vi "HEWH RLT PRAT.vi"() -> ()   [LabVIEW 2023] (continued)
            n274 = Unbundle By Name(w837) -> ("Core HEWH Data Input A.Module 4 Relay Status.Intellifaucet (% Open)"=w836:dbl, "Core HEWH Data Input A.Module 4 Relay Status.Proportioning Valve (%Open)"=w835:dbl, "Core HEWH Data Input A.Module 4 Relay Status.Intellifaucet Temp Setpoint (F)"=w834:dbl)
            n275 = local write "Valve % Open"(w836) -> ()
            n276 = local write "Proportioning\nValve"(w835) -> ()
            n277 = local write "Temp (°F)"(w834) -> ()
            n278 = call <vilib>:"Add State(s) to Queue__jki_lib_state_machine.vi"("State(s) in (\"\")"=w840) -> ("States Out"=w839:string)  [unwired: 14 in]
          }
          frame "Update File Locations" {
            n279 = flat-sequence {
              tunnel: w845 -> [w856]
              tunnel: w843 -> [w855]
              tunnel: w847 -> [w854]
              tunnel: w842 -> [w853]
              tunnel: w841 -> [w852]
              tunnel: [w851] -> w846
              tunnel: w846 -> [w857]
              tunnel: [w857] -> w844
              frame #0 {
                n280 = Bundle By Name(cluster=w856, "File Locations A"=w855, "File Locations B"=w854, "File Locations C"=w853, "File Locations D"=w852) -> (w851:T88)
              }
              frame #1 {
                n281 = Unbundle By Name(w857) -> ("Core HEWH Data Input A"=w861:T13, "Core HEWH Data Input B"=w860:T13, "Core HEWH Data Input C"=w859:T13, "Core HEWH Data Input D"=w858:T13)
                n282 = local write "Core HEWH Data Input B"(w860) -> ()
                n283 = local write "Core HEWH Data Input A"(w861) -> ()
                n284 = local write "Core HEWH Data Input C"(w859) -> ()
                n285 = local write "Core HEWH Data Input D"(w858) -> ()
              }
              frame #2 {
                "Start Draw Loop" <- TRUE ("Init Complete")
              }
            }
            n286 = call <vilib>:"Add State(s) to Queue__jki_lib_state_machine.vi"("State(s) in (\"\")"=w850) -> ("States Out"=w849:string)  [unwired: 14 in]
          }
          frame "Load Configuration" {
            w866 = u16 502 ("Test Fixture Hardware.ITHX-Temp Humidity.Remote Port")
            w875 = T89 {"Test Fixture Hardware"={"Power "={"Yokogawa"={"WT210"={"Sample Rate (1: 0.25s)"=0, "A Range (12: 20A)"=0, "V Range (6: 600V)"=0, "Power VISA Yokogawa WT210"=""}, "WT500"={"Power VISA Yokogawa WT500"="", "V Range (8: 1000V)"=0, "I Range (7: 40A)"=0, "Update Rate (3: 500ms)"=0}, "WT310_2"={"Sample Rate (1: 0.25s)"=0, "A Range (12: 20A)"=0, "V Range (6: 600V)"=0, "Power VISA Yokogawa WT310_2"=""}, "WT310_3"={"Sample Rate (1: 0.25s)"=0, "A Range (12: 20A)"=0, "V Range (6: 600V)"=0, "Power VISA Yokogawa WT310_3"=""}}, "Aplus"={"Aplus IP Address"="", "Remote Port"=0, "Instrument"="", "Instr Driver Revision"=""}, "Power Limits"={"Crest Factor"={"Upper Limit"=0.0, "Lower Limit"=0.0}, "Harmonic Content"={"Uthd"=0.0}, "Voltage"={"% Error"=0.0}, "Stability"={"<1 Watt "={"Wattage"=0.0, "Slope (mW/H)"=0.0}, ">1 Watt"={"1%Power/Hour"=0.0}}}, "Nominal Voltage"=0, "Time Limit (s)"=0.0, "Power Variation Limit (%)"=0.0, "Power Supply"={"Chroma 61605"="", "Use Chroma?"=FALSE}}, "Weight Scale"={"Com Options"={"IND560Scale VISA"="", "IP Address"="", "Remote Port"=0, "Setra Scale VISA"="", "GSE 350"=""}, "Select Scale"=""}, "Flow Rates"={"Laurel Cold IP Address"="", "Laurel Hot IP Address"="", "Hot Water Laurel VISA"="", "Cold Water Laurel VISA"="", "Remote Port"=0, "Laurel Communication Type"="", "Meters To Collect (Hot Cold)"="", "HOT Laurel Reference"=refnum, "COLD Laurel Reference"=refnum, "Modbus Hot Ref"=refnum}, "Analog Data"={"Agilent"={"Agilent 34972_1"="", "Agilent 34972_2"="", "Agilent 34972_3"="", "Agilent 34972_4"="", "Agilent 34972_5"="", "Agilent 34972_6"="", "Agilent Gain"=0.0, "TC Type (K,J,T)"="", "Instrument IDN?"="", "TC Channels-List"="", "Analog Channels-List"="", "Agilent Cluster Array"=[], "TC Channels-List 2"="", "Analog Channels-List 2"=""}, "Yokogawa"={"MW100"="", "Intellifaucet"=FALSE}, "Select Analog"="", "TC Coefficients"={"TC Coefficients 1"=[], "TC Coefficients 2"=[], "TC Coefficients 3"=[], "TC Coefficients 4"=[], "TC Coefficients 5"=[], "TC Coefficients 6"=[], "TC Coefficients 7"=[]}, "NI Tasks (Dryer DOE)"=[], "Laurel Analog"={"Laurel IP (Water Temp)"="", "Laurel IP (Pressure)"=""}}, "Viasala Temperature & Humidity"={"IP Address 1"="", "Remote Port"=0, "IP Address 2"="", "IP Address 3"="", "Viasala Modbus"=refnum, "Probe Number"=0}, "Gas Meter"={"Gas Meter 1"="", "Gas Meter 2"="", "Gas Meter 3"="", "Gas Meter 4"="", "Gas Meter 5"="", "Gas Meter 6"="", "Data Frame Format"={"Absolute Pressure"=FALSE, "Gauge/Diff. Pressure"=FALSE, "Barometric Pressure"=FALSE, "Temperature"=FALSE, "Volumetric"=FALSE, "Mass"=FALSE, "Setpoint"=FALSE, "Valve Drive"=FALSE, "Totalizer"=FALSE, "Totalizer Timer"=FALSE, "Totalizer Average Flow"=FALSE, "Totalizer Peak Flow"=FALSE, "Gas Selected"=FALSE, "Tot. Timer Format"=0}, "Measurement Units"={"Software Rev"="", "Model Number"="", "Manufacturer Info"="", "Software Sub-Rev"="", "Board Rev"="", "Units of Measure Input"={"Abs. Pressure"="", "Gauge/Diff. Press."="", "Barometric Press."="", "Temperature"="", "Volume"="", "Mass"="", "Setpoint"="", "Valve Drive"="", "Totalizer"="", "Tot. Timer"="", "Tot. Avg. Flow"="", "Tot. Peak Flow"=""}}, "Ritter Gas Meter 1"=""}, "Barometric Pressure"={"HEISE 901A"="", "Use Barometer?"=FALSE}, "Gas Analysis"={"Ultramat 23 VISA"=""}, "Inficon Micro GC"={"Propane IP Address"="192.168.1.33", "Natural Gas  IP Address"="192.168.1.32", "Remote Port"=502, "Natural Modbus"=refnum, "Propane Modbus"=refnum}, "Tenney Environmental Chamber"={"Remote Port"=0, "IP Address"="", "Tenney Modbus"=refnum}}, "GEA2"={"Address"=0, "Source"=0, "Viper/Hawk"=0}, "DOE Capacity Measurments"={"Weight 1"=0.0, "Model Number 1"="", "Temp 1"=0.0, "Serial Number 1"="", "Lab Number 1"="", "Lab Number 2"="", "Serial Number 2"="", "Temp 2"=0.0, "Model Number 2"="", "Weight 2"=0.0, "Lab Number 3"="", "Serial Number 3"="", "Temp 3"=0.0, "Model Number 3"="", "Weight 3"=0.0, "Lab Number 4"="", "Serial Number 4"="", "Temp 4"=0.0, "Model Number 4"="", "Weight 4"=0.0, "Capacity Measurment Output String"=[]}, "Initialize.Washer In"={"Appliance Details"={"FileVersionInfo"={"FileVersion"="", "ProductName"="", "InternalName"="", "CompanyName"="", "LegalCopyright"="", "FileDescription"=""}, "Dishwasher Info"={"Open Cup Weight (gm):"=0.0, "Auto Cup Weight (gm):"=0.0, "Detergent-Dish:"="", "Inlet Temperature-Dish:"="", "Cycle Mode-Dish:"="", "Unit Control-Dish:"="", "Manufacturer-Dish:"=""}, "Washer Info"={"Hot Water Temperature (Fahrenheit):"="", "Cold Water Temperature (Fahrenheit):"="", "Capacity (cu.ft):"=0.0, "Initial Cloth Weight:"=0.0, "Cloth Lot:"=0, "Model Family:"="", "Program Name:"="", "Cycle Selection:"="", "Wash Temperature:"="", "Rinse Temperature:"="", "Load Size:"=""}, "File Name Output Array"=[], "Calibration Output Array"=[], "Appliance Common"={"Engineer:"="", "Model Number:"="", "Serial Number:"="", "Comments:"="", "Station ID:"="", "Technician:"="", "TR Number:"="", "Lab ID:"="", "Voltage:"="", "Water Pressure (PSI):"="", "Test Date:"="", "Computer Name:"="", "IP Address:"="", "Ambient RH:"="", "Frequency:"="", "Build:"="", "Filename:"="", "Test Type:"="", "Load Run #:"=0, "Ambient Temperature (F):"="", "File Path:"=path "", "Cycles Per Year"=0}, "Water Heater"={"Heating Mode:"=""}, "Dryer"={"Heat Setting:"="", "Washer Water Temperature (60 ± 5°F):"=0, "Water Hardness (PPM):"=0, "Dryness Setting:"="", "Dryer Type:"="", "Exhaust:"="", "Drying Cycle:"="", "Load Type:"="", "Nominal Load Weight"="", "Dryer Initial IMC Data"={"Measured IMC (lbs)"=0.0, "Actual Initial RMC (%)"=0.0, "RMC (Desired %)"=0.0, "Bone Dry Wt(lbs)"=0.0, "Tolerance(%)"=0.0, "Actual Final RMC (%)"=0.0, "CEF (lbf/kWh)"=0.0, "Minimum Weight (lbf)"=0.0, "Average Weight (lbf)"=0.0, "Maximum Weight (lbf)"=0.0, "Measured IMC In Range?"=FALSE, "Moisture Reduction Factor"=0.0, "Field Use Factor"=0.0, "Empty Dryer Cold Weigth"=0.0, "Energy Standard"=enum."D2-Automatic Dryer", "Weight Cloth (lbs)"=0.0, "Relative Moisture Content (%)"=0.0, "Relative Moisture Content - Avg (%)"=0.0}}}, "Display Data (RLT)"={"Status Color"=0, "Serial Number Display"="", "Cycle Count Display"=0, "Station Label Display"="", "Current Run Start Time Display"=0.0, "Board ID Display"="", "RPM Display"=0, "Current Display"=0.0, "Current Path Display"=path "", "Saving Display"=FALSE, "Unit Type Display"=enum."", "Total Time On Display"=0.0, "UI Button"=FALSE}}} ("Washer Controls In")
            w876 = Save_File_DOE_Configuration_State."Load Config" ("Config State")
            # "IP Address = Tenney IP Address\nIP Address 1 = Viasala IP Address"
            n287 = flat-sequence {
              frame #0 {
                w903 = FALSE ("GEA2_A?")
                n288 = local write "GEA2_B?"(w903) -> ()
                n289 = local write "GEA2_A?"(w903) -> ()
                n290 = local write "GEA2_C?"(w903) -> ()
                n291 = local write "GEA2_D?"(w903) -> ()
              }
              frame #1 {
                w904 = T87."Disabled and Grayed Out" ("Disabled")
                n292 = property on="Update User Setpoint" class="Bool"("DisabledEnum"=w904) -> ()  [unwired: 2 in, 2 out]
                n293 = property on="Update Mode" class="Bool"("DisabledEnum"=w904) -> ()  [unwired: 2 in, 2 out]
                n294 = property on="Update TankSP Offset" class="Bool"("DisabledEnum"=w904) -> ()  [unwired: 2 in, 2 out]
                n295 = property on="Update Personality" class="Bool"("DisabledEnum"=w904) -> ()  [unwired: 2 in, 2 out]
              }
            }
            n296 = Unbundle By Name(w882) -> ("Core HEWH Data Input A.LV Program"=w871:T25, "File Locations A"=w884:T3, "File Locations B"=w874:T3, "File Locations C"=w873:T3, "File Locations D"=w872:T3)
            n297 = call "Save File DOE File Setup.vi"("Filepath In"=w884, "Washer Controls In"=w875, "error in (no error)"=w885, "Config State"=w876, "LV Program"=w871) -> ("Washer Controls Out"=w883:T89, "Filepath Out"=w867:T3, "error out"=w878:errorcluster)  [unwired: 12 in]
            n298 = Unbundle By Name(w883) -> ("Test Fixture Hardware.Tenney Environmental Chamber.IP Address"=w865:string, "Test Fixture Hardware.Viasala Temperature & Humidity.IP Address 1"=w864:string, "Test Fixture Hardware.Viasala Temperature & Humidity.Probe Number"=w863:u16, "Test Fixture Hardware.Flow Rates.Laurel Hot IP Address"=w881:string, "Test Fixture Hardware.Flow Rates.Laurel Cold IP Address"=w879:string)
            "Laurel Cold IP Address" <- w879
            "Viasala.Probe Number" <- w863
            n299 = case shown="\"PRAT\", \"HEWH RLT\"" w871 {
              tunnel: w878 -> [w889 w902]
              tunnel: [w889 w899] -> w877
              tunnel: w876 -> [_ w898]
              tunnel: w871 -> [_ w897]
              tunnel: w875 -> [_ w896]
              tunnel: w874 -> [_ w895]
              tunnel: w873 -> [_ w894]
              tunnel: w872 -> [_ w893]
              tunnel: [w888 w892] -> w870
              tunnel: [w888 w891] -> w869
              tunnel: [w888 w890] -> w868
              tunnel: w867 -> [w888 _]
              frame Default {
              }
              frame "PRAT", "HEWH RLT" {
                n300 = call "Save File DOE File Setup.vi"("Filepath In"=w895, "Washer Controls In"=w896, "error in (no error)"=w902, "Config State"=w898, "LV Program"=w897) -> ("Filepath Out"=w892:T3, "error out"=w901:errorcluster)  [unwired: 12 in, 1 out]
                n301 = call "Save File DOE File Setup.vi"("Filepath In"=w894, "Washer Controls In"=w896, "error in (no error)"=w901, "Config State"=w898, "LV Program"=w897) -> ("Filepath Out"=w891:T3, "error out"=w900:errorcluster)  [unwired: 12 in, 1 out]
                n302 = call "Save File DOE File Setup.vi"("Filepath In"=w893, "Washer Controls In"=w896, "error in (no error)"=w900, "Config State"=w898, "LV Program"=w897) -> ("Filepath Out"=w890:T3, "error out"=w899:errorcluster)  [unwired: 12 in, 1 out]
              }
            }
            n303 = call <vilib>:"Add State(s) to Queue__jki_lib_state_machine.vi"("State(s) in (\"\")"=w887) -> ("States Out"=w886:string)  [unwired: 14 in]
            n304 = Bundle By Name(cluster=w882, "Test Fixture Hardware.Tenney Environmental Chamber.IP Address"=w865, "Test Fixture Hardware.Tenney Environmental Chamber.Remote Port"=w866, "Test Fixture Hardware.Viasala Temperature & Humidity.Remote Port"=w866, "Test Fixture Hardware.Viasala Temperature & Humidity.IP Address 1"=w864, "Test Fixture Hardware.Viasala Temperature & Humidity.Probe Number"=w863, "Test Fixture Hardware.Flow Rates.Laurel Hot IP Address"=w881, "Test Fixture Hardware.Flow Rates.Laurel Cold IP Address"=w879, "File Locations A"=w867, "File Locations B"=w870, "File Locations C"=w869, "File Locations D"=w868) -> (w880:T88)
          }
          frame "Init Hot Laurel" {
            n305 = Unbundle By Name(w905) -> ("Test Fixture Hardware.Flow Rates.Laurel Cold IP Address"=w908:string, "Test Fixture Hardware.Flow Rates.Laurel Hot IP Address"=w907:string, "Test Fixture Hardware.Flow Rates.Laurel Cold IP Address"=w909:string)
            n306 = call "HEWH Select Master Flow Meter.vi"("Laurel Hot IP Address"=w907, "Laurel Cold IP Address"=w908) -> ("Flow Selector"=w906:T93)  [unwired: 7 in, 2 out]
            n307 = case shown="\"Hot\"" w906 {
              tunnel: w911 -> [w914 w915 w917 w919]
              tunnel: [w914 w915 w917 w919] -> w910
              tunnel: w909 -> [_ _ _ _]
              tunnel: w907 -> [_ _ _ _]
              frame "None", Default {
              }
              frame "Hot and Cold" {
                n308 = property on="Reset Inventory" class="Bool"("DisabledEnum"=T87."Enabled" ("Disabled")) -> ()  [unwired: 2 in, 2 out]
              }
              frame "Hot" {
                n309 = property on="Reset Inventory" class="Bool"("DisabledEnum"=T87."Disabled and Grayed Out" ("Disabled")) -> ()  [unwired: 2 in, 2 out]
              }
              frame "Cold" {
                n310 = property on="Reset Inventory" class="Bool"("DisabledEnum"=T87."Enabled" ("Disabled")) -> ()  [unwired: 2 in, 2 out]
              }
            }
            n311 = call <vilib>:"Add State(s) to Queue__jki_lib_state_machine.vi"("State(s) in (\"\")"=w913) -> ("States Out"=w912:string)  [unwired: 14 in]
          }
          frame "DAQ Loop Complete" {
            w921 = TRUE ("Init Complete")
            n312 = Unbundle By Name(w927) -> ("Test Fixture Hardware"=→"Test Fixture Hardware Draw Loop":T55)
            n313 = call <vilib>:"Add State(s) to Queue__jki_lib_state_machine.vi"("State(s) in (\"\")"=w929) -> ("States Out"=w928:string)  [unwired: 14 in]
            n314 = call "UTILITY Boolean Notifier.vi"("Status"=UTILITY_Notifier."Set", "error in (no error)"=w923, "Set Status"=w921, "name (unnamed)"="Splash") -> ("error out"=w922:errorcluster)  [unwired: 6 in, 1 out]
            "DAQ Complete" <- w921
          }
          frame "Shutdown Equipment" {
            n315 = Unbundle By Name(w936) -> ("Test Fixture Hardware"=w931:T55, "Core HEWH Data Input A"=w935:T13)
            n316 = local read "Pressurize Tank?"() -> (w932:bool)
            n317 = call "HEWH Close Equipmet.vi"("Test Fixture Hardware In"=w931, "Pressurize Tank"=w932, "Core HEWH Data"=w935, "Error In"=w934, "Refnum in"=w933) -> ("Error Out"=w930:errorcluster)  [unwired: 8 in, 2 out]
            n318 = call <vilib>:"Add State(s) to Queue__jki_lib_state_machine.vi"("State(s) in (\"\")"=w938) -> ("States Out"=w937:string)  [unwired: 14 in]
          }
          frame "---------- Data ----------" {
            n319 = call <vilib>:"Add State(s) to Queue__jki_lib_state_machine.vi"("State(s) in (\"\")"=w942) -> ("States Out"=w941:string)  [unwired: 14 in]
          }
          frame "Data: Get Time" {
            w952 = string[][] [] ("A Data Array")
            # "allows reset after purge"
            # "Reset Array"
            n320 = Bundle By Name(cluster=w950, "A Data Array"=w952, "B Data Array"=w952, "C Data Array"=w952, "D Data Array"=w952) -> (w951:T88)
            n321 = local read item#-1() -> (w944)
            n322 = case shown="\"Four Stations\"" w949 {
              tunnel: [w958 w959] -> w945
              tunnel: [w958 w960] -> w946
              tunnel: [w958 w961] -> w947
              tunnel: [w956 w962] -> w948
              tunnel: w944 -> [w957 w963]
              frame "Single Station", Default {
                w958 = string[][] [] ("Total Array")
                n323 = Unbundle By Name(w957) -> ("Station A-Timer"=w956)
              }
              frame "Four Stations" {
                n324 = Unbundle By Name(w963) -> ("Station A-Timer"=w962, "Station B-Timer"=w961, "Station C-Timer"=w960, "Station D-Timer"=w959)
              }
            }
            n325 = call <vilib>:"Add State(s) to Queue__jki_lib_state_machine.vi"("State(s) in (\"\")"=w955) -> ("States Out"=w954:string)  [unwired: 14 in]
            n326 = Bundle By Name(cluster=w951, "A Data Array"=w948, "B Data Array"=w947, "C Data Array"=w946, "D Data Array"=w945) -> (w953:T88)
          }
          frame "Data: Get MW100 (Station A)" {
            w978 = "A" ("Prat Station")
            n327 = Unbundle By Name(w1000) -> ("A Data Array"=w1002:string[][], "Test Fixture Hardware"=w964:T55, "Core HEWH Data Input A"=w994:T13, "RLT Station Channels.MW100.Station A Channels, MW100"=w980:string[][])
            n328 = call "UTILITY Aquire Semaphore.vi"("error in (no error)"=w997, "Refnum in"=w996) -> ("error out"=w998:errorcluster, "Refnum out"=w999:T83)  [unwired: 8 in]
            n329 = local read "Draw Station"() -> (w992:string)
            n330 = property on="Cycle Count Display" class="DigNum (strict)"() -> ("Value"=w989:i32)  [unwired: 2 in, 2 out]
            n331 = call "HEWH Gather Test Data.vi"("Test Fixture Hardware Input"=w964, "Core HEWH Data Station A"=w994, "GEA2?"="GEA2_A?", "error in (no error)"=w998, "Station ID"=w978, "Draw Count"=w989, "Disable Relay Check During Draw?"=FALSE) -> ("Core HEWH Data Station A"=w967:T13, "Emerson Flow Meter Data Output"=w966:T72, "MW100 Full Data"=w979:string[][], "error out"=w987:errorcluster)  [unwired: 7 in, 2 out]
            n332 = call "HEWH RLT Selected MW100 TCs.vi"("Core HEWH Data Station A"=w967, "Current Drawing Station"=w992, "Show Flow Data"="Show Stand Override Flow Data A", "MW100 Full Data"=w979, "Error In"=w987, "Station A Channels, MW100"=w980, "Station ID"=w978, "Collect Power Data"="DAQ for A") -> ("Data (Label,Data)"=w983:string[][], "Core HEWH Data Station Output"=w982:T13, "RMS Current (Amps)"=w993:dbl, "TC Data"=w985:string[][], "Error Out"=w991:errorcluster)  [unwired: 3 in]
            n333 = call "HEWH Tank Display.vi"("Core HEWH Data Station A"=w982, "TC Data"=w985, "error in"=w991, "Station ID"=w978, "DAQ for A"="DAQ for A") -> ("Core HEWH Data Station Output"=w975:T13, "Tank Display - Station A"=→"Tank Display - Station A":T36, "error out"=w968:errorcluster)  [unwired: 8 in]
            n334 = Build Array (concatenate)(w1002, w983) -> (w1001:string[][])
            n335 = Unbundle By Name(w975) -> ("Module 4 Relay Status"=→"Module 4 Relay Status":T28, "LV Program"=w990:T25)
            n336 = local read "Test CompleteA"() -> (w976:bool)
            n337 = call "HEWH MW100 Data.vi"("Status"=UTILITY_Notifier."Set", "error in (no error)"=w968, "Core HEWH Data Input A"=w967, "name (unnamed)"="MW100") -> ("error out"=w973:errorcluster)  [unwired: 6 in, 1 out]
            n338 = case shown="\"HEWH\"" w990 {
              tunnel: w993 -> [_ w1006 w1007]
              frame Default {
              }
              frame "PRAT" {
                "Current (A)" <- w1006
              }
              frame "HEWH" {
                n339 = local write "Current (A)"(w1007) -> ()
              }
            }
            n340 = Bundle By Name(cluster=w1000, "Core HEWH Data Input A.Test Complete"=w976, "A Data Array"=w1001, "Core HEWH Data Input A"=w975) -> (w1003:T88)
            n341 = call "HEWH Emerson Data.vi"("Status"=UTILITY_Notifier."Set", "error in (no error)"=w973, "Emerson Flow Meter Data Input"=w966, "name (unnamed)"="Emerson") -> ("error out"=w965:errorcluster)  [unwired: 6 in, 1 out]
            n342 = call <vilib>:"Add State(s) to Queue__jki_lib_state_machine.vi"("State(s) in (\"\")"=w1005) -> ("States Out"=w1004:string)  [unwired: 14 in]
            n343 = call "UTILITY Release Semaphore.vi"("error in (no error)"=w965, "Refnum in"=w999) -> ("error out"=w995:errorcluster)  [unwired: 9 in]
          }
          frame "Data: Get MW100 (Station B)" {
            w1012 = "B" ("Prat Station")
            n344 = Unbundle By Name(w1038) -> ("B Data Array"=w1030:string[][], "Test Fixture Hardware"=w1016:T55, "Core HEWH Data Input B"=w1032:T13, "RLT Station Channels.MW100.Station B Channels, MW100"=w1027:string[][])
            n345 = property on="Cycle Count Display" class="DigNum (strict)"() -> ("Value"=w1022:i32)  [unwired: 2 in, 2 out]
            n346 = call "UTILITY Aquire Semaphore.vi"("error in (no error)"=w1035, "Refnum in"=w1034) -> ("error out"=w1036:errorcluster, "Refnum out"=w1037:T83)  [unwired: 8 in]
            n347 = call "HEWH Gather Test Data.vi"("Test Fixture Hardware Input"=w1016, "Core HEWH Data Station A"=w1032, "GEA2?"="GEA2_B?", "error in (no error)"=w1036, "Station ID"=w1012, "Draw Count"=w1022, "Disable Relay Check During Draw?"=FALSE) -> ("Core HEWH Data Station A"=w1013:T13, "MW100 Full Data"=w1017:string[][], "error out"=w1028:errorcluster)  [unwired: 7 in, 3 out]
            n348 = local read "Draw Station"() -> (w1025:string)
            n349 = call "HEWH RLT Selected MW100 TCs.vi"("Core HEWH Data Station A"=w1013, "Current Drawing Station"=w1025, "Show Flow Data"="Show Stand Override Flow Data B", "MW100 Full Data"=w1017, "Error In"=w1028, "Station A Channels, MW100"=w1027, "Station ID"=w1012, "Collect Power Data"="DAQ for B") -> ("Data (Label,Data)"=w1029:string[][], "Core HEWH Data Station Output"=w1009:T13, "RMS Current (Amps)"=w1026:dbl, "TC Data"=w1010:string[][], "Error Out"=w1024:errorcluster)  [unwired: 3 in]
            n350 = Build Array (concatenate)(w1030, w1029) -> (w1031:string[][])
            n351 = call "HEWH Tank Display.vi"("Core HEWH Data Station A"=w1009, "TC Data"=w1010, "error in"=w1024, "Station ID"=w1012, "DAQ for A"="DAQ for B") -> ("Core HEWH Data Station Output"=w1008:T13, "Tank Display - Station A"=→"Tank Display - Station B":T36, "error out"=w1023:errorcluster)  [unwired: 8 in]
            n352 = Unbundle By Name(w1008) -> ("LV Program"=w1015:T25)
            n353 = case shown="\"HEWH\"" w1015 {
              tunnel: w1026 -> [_ w1042 w1043]
              frame Default {
              }
              frame "PRAT" {
                "Current (B)" <- w1042
              }
              frame "HEWH" {
                n354 = local write "Current (B)"(w1043) -> ()
              }
            }
            n355 = local read "Test CompleteB"() -> (w1019:bool)
            n356 = call "UTILITY Release Semaphore.vi"("error in (no error)"=w1023, "Refnum in"=w1037) -> ("error out"=w1033:errorcluster)  [unwired: 9 in]
            n357 = Bundle By Name(cluster=w1038, "B Data Array"=w1031, "Core HEWH Data Input B.Test Complete"=w1019, "Core HEWH Data Input B"=w1008) -> (w1039:T88)
            n358 = call <vilib>:"Add State(s) to Queue__jki_lib_state_machine.vi"("State(s) in (\"\")"=w1041) -> ("States Out"=w1040:string)  [unwired: 14 in]
          }
          frame "Data: Get MW100 (Station C)" {
            w1051 = "C" ("Prat Station")
            n359 = Unbundle By Name(w1074) -> ("C Data Array"=w1066:string[][], "Test Fixture Hardware"=w1052:T55, "Core HEWH Data Input C"=w1068:T13, "RLT Station Channels.MW100.Station C Channels, MW100"=w1063:string[][])
            n360 = call "UTILITY Aquire Semaphore.vi"("error in (no error)"=w1071, "Refnum in"=w1070) -> ("error out"=w1072:errorcluster, "Refnum out"=w1073:T83)  [unwired: 8 in]
            n361 = property on="Cycle Count Display" class="DigNum (strict)"() -> ("Value"=w1058:i32)  [unwired: 2 in, 2 out]
            n362 = local read "Draw Station"() -> (w1061:string)
            n363 = call "HEWH Gather Test Data.vi"("Test Fixture Hardware Input"=w1052, "Core HEWH Data Station A"=w1068, "GEA2?"="GEA2_C?", "error in (no error)"=w1072, "Station ID"=w1051, "Draw Count"=w1058, "Disable Relay Check During Draw?"=FALSE) -> ("Core HEWH Data Station A"=w1049:T13, "MW100 Full Data"=w1053:string[][], "error out"=w1065:errorcluster)  [unwired: 7 in, 3 out]
            n364 = call "HEWH RLT Selected MW100 TCs.vi"("Core HEWH Data Station A"=w1049, "Current Drawing Station"=w1061, "Show Flow Data"="Show Stand Override Flow Data C", "MW100 Full Data"=w1053, "Error In"=w1065, "Station A Channels, MW100"=w1063, "Station ID"=w1051, "Collect Power Data"="DAQ for C") -> ("Data (Label,Data)"=w1064:string[][], "Core HEWH Data Station Output"=w1048:T13, "RMS Current (Amps)"=w1062:dbl, "TC Data"=w1047:string[][], "Error Out"=w1060:errorcluster)  [unwired: 3 in]
            n365 = Build Array (concatenate)(w1066, w1064) -> (w1067:string[][])
            n366 = call "HEWH Tank Display.vi"("Core HEWH Data Station A"=w1048, "TC Data"=w1047, "error in"=w1060, "Station ID"=w1051, "DAQ for A"="DAQ for C") -> ("Core HEWH Data Station Output"=w1044:T13, "Tank Display - Station A"=→"Tank Display - Station C":T36, "error out"=w1059:errorcluster)  [unwired: 8 in]
            n367 = Unbundle By Name(w1044) -> ("LV Program"=w1050:T25)
            n368 = local read "Test CompleteC"() -> (w1055:bool)
            n369 = case shown="\"HEWH\"" w1050 {
              tunnel: w1062 -> [_ w1078 w1079]
              frame Default {
              }
              frame "PRAT" {
                "Current (C)" <- w1078
              }
              frame "HEWH" {
                n370 = local write "Current (C)"(w1079) -> ()
              }
            }
            n371 = call "UTILITY Release Semaphore.vi"("error in (no error)"=w1059, "Refnum in"=w1073) -> ("error out"=w1069:errorcluster)  [unwired: 9 in]
            n372 = Bundle By Name(cluster=w1074, "C Data Array"=w1067, "Core HEWH Data Input C.Test Complete"=w1055, "Core HEWH Data Input C"=w1044) -> (w1075:T88)
            n373 = call <vilib>:"Add State(s) to Queue__jki_lib_state_machine.vi"("State(s) in (\"\")"=w1077) -> ("States Out"=w1076:string)  [unwired: 14 in]
          }
          frame "Data: Get MW100 (Station D)" {
            w1088 = "D" ("Prat Station")
            n374 = Unbundle By Name(w1110) -> ("D Data Array"=w1102:string[][], "Test Fixture Hardware"=w1085:T55, "Core HEWH Data Input D"=w1104:T13, "RLT Station Channels.MW100.Station D Channels, MW100"=w1101:string[][])
            n375 = local read "Draw Station"() -> (w1097:string)
            n376 = property on="Cycle Count Display" class="DigNum (strict)"() -> ("Value"=w1094:i32)  [unwired: 2 in, 2 out]
            n377 = call "UTILITY Aquire Semaphore.vi"("error in (no error)"=w1107, "Refnum in"=w1106) -> ("error out"=w1108:errorcluster, "Refnum out"=w1109:T83)  [unwired: 8 in]
            n378 = call "HEWH Gather Test Data.vi"("Test Fixture Hardware Input"=w1085, "Core HEWH Data Station A"=w1104, "GEA2?"="GEA2_D?", "error in (no error)"=w1108, "Station ID"=w1088, "Draw Count"=w1094, "Disable Relay Check During Draw?"=FALSE) -> ("Core HEWH Data Station A"=w1081:T13, "MW100 Full Data"=w1089:string[][], "error out"=w1100:errorcluster)  [unwired: 7 in, 3 out]
            n379 = call "HEWH RLT Selected MW100 TCs.vi"("Core HEWH Data Station A"=w1081, "Current Drawing Station"=w1097, "Show Flow Data"="Show Stand Override Flow Data D", "MW100 Full Data"=w1089, "Error In"=w1100, "Station A Channels, MW100"=w1101, "Station ID"=w1088, "Collect Power Data"="DAQ for D") -> ("Data (Label,Data)"=w1099:string[][], "Core HEWH Data Station Output"=w1082:T13, "RMS Current (Amps)"=w1098:dbl, "TC Data"=w1083:string[][], "Error Out"=w1096:errorcluster)  [unwired: 3 in]
            n380 = call "HEWH Tank Display.vi"("Core HEWH Data Station A"=w1082, "TC Data"=w1083, "error in"=w1096, "Station ID"=w1088, "DAQ for A"="DAQ for D") -> ("Core HEWH Data Station Output"=w1080:T13, "Tank Display - Station A"=→"Tank Display - Station D":T36, "error out"=w1095:errorcluster)  [unwired: 8 in]
            n381 = Build Array (concatenate)(w1102, w1099) -> (w1103:string[][])
            n382 = Unbundle By Name(w1080) -> ("LV Program"=w1084:T25)
            n383 = local read "Test CompleteD"() -> (w1091:bool)
            n384 = case shown="\"HEWH\"" w1084 {
              tunnel: w1098 -> [_ w1114 w1115]
              frame Default {
              }
              frame "PRAT" {
                "Current (D)" <- w1114
              }
              frame "HEWH" {
                n385 = local write "Current (D)"(w1115) -> ()
              }
            }
            n386 = call "UTILITY Release Semaphore.vi"("error in (no error)"=w1095, "Refnum in"=w1109) -> ("error out"=w1105:errorcluster)  [unwired: 9 in]
            n387 = call <vilib>:"Add State(s) to Queue__jki_lib_state_machine.vi"("State(s) in (\"\")"=w1113) -> ("States Out"=w1112:string)  [unwired: 14 in]
            n388 = Bundle By Name(cluster=w1110, "D Data Array"=w1103, "Core HEWH Data Input D.Test Complete"=w1091, "Core HEWH Data Input D"=w1080) -> (w1111:T88)
          }
          frame "Data: Get GEA2 A" {
            # "This will need to be the \"Coldest Day\" ERD"
            # "If no GEA...you still need to \nfill in the elements into data \narray"
            # "Get the Bus Data. This is data from the actual unit"
            n389 = Unbundle By Name(w1129) -> ("A Data Array"=w1139:string[][], "Core HEWH Data Input A.HEWH Specific DAQ"=w1127:T21)
            n390 = local read item#-1() -> (w1118)
            n391 = local read "GEA2_A?"() -> ()  [unwired: 1 out]
            n392 = local read item#-1() -> (w1121)
            n393 = Unbundle By Name(w1118) -> ("ERD Data Input"=w1117, "ERD Data"=w1116)
            n394 = local read "GEA2_A?"() -> (w1125:bool)
            n395 = local read item#-1() -> (w1120)
            n396 = local read "Vesta Data Output"() -> (w1126:T66)
            n397 = local read item#-1() -> (w1123)
            n398 = Unbundle By Name(w1120) -> ("Data Cluster"=w1119)
            n399 = Or(x=w1125, y=w1121) -> (x .or. y?=w1124:bool)
            n400 = Or(x=w1123, y=w1121) -> (x .or. y?=w1122:bool)
            n401 = call "HEWH Build String Diagnostics Data.vi"("GEA2"=w1124, "Pilot (SCFH)"="Pilot Flow Rate (SCFH)", "ERD Data  2"=w1117, "Vesta Data Output"=w1126, "ERD Data"=w1116, "Get Gas Data"=w1122, "Measurement Data"=w1119, "HEWH Specific DAQ"=w1127) -> ("Power Display"=w1132:T23, "Appliance Data"=w1131:string[][], "Error Out"=w1128:errorcluster)  [unwired: 5 in]
            "POWERA" <- w1132
            "POWERA Display" <- w1132
            n402 = call <vilib>:"Add State(s) to Queue__jki_lib_state_machine.vi"("State(s) in (\"\")"=w1136) -> ("States Out"=w1137:string)  [unwired: 14 in]
            n403 = call "HEWH Power Notifier.vi"("Status"=UTILITY_Notifier."Set", "Set Status"=w1132, "name (unnamed)"="PowerA") -> ()  [unwired: 7 in, 2 out]
            n404 = Build Array (concatenate)(w1139, w1131) -> (w1138:string[][])
            n405 = Bundle By Name(cluster=w1129, "A Data Array"=w1138) -> (w1135:T88)
          }
          frame "Data: Get GEA2 B" {
            # "Get the Bus Data"
            n406 = Unbundle By Name(w1151) -> ("B Data Array"=w1156:string[][], "Core HEWH Data Input B.HEWH Specific DAQ"=w1143:T21)
            n407 = local read "GEA2_B?"() -> ()  [unwired: 1 out]
            n408 = local read "GEA2_B?"() -> (w1144:bool)
            n409 = local read item#-1() -> (w1142)
            n410 = local read item#-1() -> (w1141)
            n411 = call "HEWH Build String Diagnostics Data.vi"("GEA2"=w1144, "ERD Data  2"=w1142, "ERD Data"=w1141, "Error In"=w1140, "Get Gas Data"=FALSE ("Disable Classic GEA2"), "HEWH Specific DAQ"=w1143) -> ("Power Display"=w1146:T23, "Appliance Data"=w1147:string[][], "Error Out"=w1148:errorcluster)  [unwired: 7 in]
            "POWERB" <- w1146
            "POWERB Display" <- w1146
            n412 = call "HEWH Power Notifier.vi"("Status"=UTILITY_Notifier."Set", "Set Status"=w1146, "name (unnamed)"="PowerB") -> ()  [unwired: 7 in, 2 out]
            n413 = call <vilib>:"Add State(s) to Queue__jki_lib_state_machine.vi"("State(s) in (\"\")"=w1153) -> ("States Out"=w1154:string)  [unwired: 14 in]
            n414 = Build Array (concatenate)(w1156, w1147) -> (w1155:string[][])
            n415 = Bundle By Name(cluster=w1151, "B Data Array"=w1155) -> (w1152:T88)
          }
          frame "Data: Get GEA2 C" {
            # "Get the Bus Data"
            n416 = Unbundle By Name(w1168) -> ("C Data Array"=w1173:string[][], "Core HEWH Data Input C.HEWH Specific DAQ"=w1160:T21)
            n417 = local read "GEA2_C?"() -> ()  [unwired: 1 out]
            n418 = local read "GEA2_C?"() -> (w1161:bool)
            n419 = local read item#-1() -> (w1159)
            n420 = local read item#-1() -> (w1158)
            n421 = call "HEWH Build String Diagnostics Data.vi"("GEA2"=w1161, "ERD Data  2"=w1159, "ERD Data"=w1158, "Error In"=w1157, "Get Gas Data"=FALSE ("Disable Classic GEA2"), "HEWH Specific DAQ"=w1160) -> ("Power Display"=w1164:T23, "Appliance Data"=w1163:string[][], "Error Out"=w1165:errorcluster)  [unwired: 7 in]
            "POWERC" <- w1164
            "POWERC Display" <- w1164
            n422 = call "HEWH Power Notifier.vi"("Status"=UTILITY_Notifier."Set", "Set Status"=w1164, "name (unnamed)"="PowerC") -> ()  [unwired: 7 in, 2 out]
            n423 = call <vilib>:"Add State(s) to Queue__jki_lib_state_machine.vi"("State(s) in (\"\")"=w1170) -> ("States Out"=w1171:string)  [unwired: 14 in]
            n424 = Build Array (concatenate)(w1173, w1163) -> (w1172:string[][])
            n425 = Bundle By Name(cluster=w1168, "C Data Array"=w1172) -> (w1169:T88)
          }
          frame "Data: Get GEA2 D" {
            # "Get the Bus Data"
            n426 = Unbundle By Name(w1185) -> ("D Data Array"=w1190:string[][], "Core HEWH Data Input D.HEWH Specific DAQ"=w1177:T21)
            n427 = local read "GEA2_D?"() -> ()  [unwired: 1 out]
            n428 = local read "GEA2_D?"() -> (w1178:bool)
            n429 = local read item#-1() -> (w1175)
            n430 = local read item#-1() -> (w1174)
            n431 = call "HEWH Build String Diagnostics Data.vi"("GEA2"=w1178, "ERD Data  2"=w1175, "ERD Data"=w1174, "Error In"=w1176, "Get Gas Data"=FALSE, "HEWH Specific DAQ"=w1177) -> ("Power Display"=w1181:T23, "Appliance Data"=w1180:string[][], "Error Out"=w1182:errorcluster)  [unwired: 7 in]
            "POWERD" <- w1181
            "POWERD Display" <- w1181
            n432 = call "HEWH Power Notifier.vi"("Status"=UTILITY_Notifier."Set", "Set Status"=w1181, "name (unnamed)"="PowerD") -> ()  [unwired: 7 in, 2 out]
            n433 = call <vilib>:"Add State(s) to Queue__jki_lib_state_machine.vi"("State(s) in (\"\")"=w1187) -> ("States Out"=w1188:string)  [unwired: 14 in]
            n434 = Build Array (concatenate)(w1190, w1180) -> (w1189:string[][])
            n435 = Bundle By Name(cluster=w1185, "D Data Array"=w1189) -> (w1186:T88)
          }
          frame "Data: Get Agilent" {
            # "Acquire Agilent Data"
            n436 = Unbundle By Name(w1196) -> ("A Data Array"=w1200:string[][], "B Data Array"=w1199:string[][], "C Data Array"=w1198:string[][], "D Data Array"=w1197:string[][])
            n437 = local read item#-1() -> ()  [unwired: 1 out]
            n438 = call <vilib>:"Add State(s) to Queue__jki_lib_state_machine.vi"("State(s) in (\"\")"=w1203) -> ("States Out"=w1202:string)  [unwired: 14 in]
            n439 = Build Array (concatenate)(w1200) -> (w1195:string[][])  [unwired: 1 in]
            n440 = Build Array (concatenate)(w1199) -> (w1194:string[][])  [unwired: 1 in]
            n441 = Build Array (concatenate)(w1198) -> (w1193:string[][])  [unwired: 1 in]
            n442 = Build Array (concatenate)(w1197) -> (w1192:string[][])  [unwired: 1 in]
            n443 = Bundle By Name(cluster=w1196, "A Data Array"=w1195, "B Data Array"=w1194, "C Data Array"=w1193, "D Data Array"=w1192) -> (w1201:T88)
          }
          frame "Get Temp and Humidity" {
            # "Acquire Temp/Humidity Data"
            n444 = Unbundle By Name(w1213) -> ("Test Fixture Hardware.Viasala Temperature & Humidity.Probe Number"=w1204:u16, "A Data Array"=w1217:string[][], "B Data Array"=w1216:string[][], "C Data Array"=w1215:string[][], "D Data Array"=w1214:string[][], "Core HEWH Data Input A.LV Program"=w1208:T25)
            n445 = local read item#-1() -> ()  [unwired: 1 out]
            n446 = call "Viasala Indigo 520-String Data.vi"("error in (no error)"=w1206, "Viasala Probe Number"=w1204) -> ("error out"=w1207:errorcluster, "Viasala Data"=w1205:string[][])  [unwired: 7 in, 1 out]
            n447 = case shown="Default" w1208 {
              tunnel: w1217 -> [w1221 w1230]
              tunnel: w1216 -> [w1225 w1229]
              tunnel: w1215 -> [w1224 w1228]
              tunnel: w1214 -> [w1223 w1227]
              tunnel: [w1226 w1230] -> w1212
              tunnel: [w1225 w1229] -> w1211
              tunnel: [w1224 w1228] -> w1210
              tunnel: [w1223 w1227] -> w1209
              tunnel: w1205 -> [w1222 _]
              frame Default {
                n448 = Build Array (concatenate)(w1221, w1222) -> (w1226:string[][])
              }
              frame "PRAT", "HEWH RLT" {
              }
            }
            n449 = Bundle By Name(cluster=w1213, "A Data Array"=w1212, "B Data Array"=w1211, "C Data Array"=w1210, "D Data Array"=w1209) -> (w1218:T88)
            n450 = call <vilib>:"Add State(s) to Queue__jki_lib_state_machine.vi"("State(s) in (\"\")"=w1220) -> ("States Out"=w1219:string)  [unwired: 14 in]
          }
          frame "Get HHV" {
            # "Acquire Inficon Heating Value Data"
            n451 = Unbundle By Name(w1238) -> ("Core HEWH Data Input A.LV Program"=w1237:T25)
            n452 = local read item#-1() -> (w1232)
            n453 = local read item#-1() -> (w1235)
            n454 = local read item#-1() -> (w1234)
            n455 = Unbundle By Name(w1232) -> ("Data Cluster.Gas selected"=w1231)
            n456 = call <vilib>:"Add State(s) to Queue__jki_lib_state_machine.vi"("State(s) in (\"\")"=w1245) -> ("States Out"=w1244:string)  [unwired: 14 in]
            n457 = case shown="\"CH4\", \"NatG-1\", \"NatG-2\", \"NatG-3\"" w1231 {
              tunnel: w1243 -> [w1253 w1256 w1280]
              tunnel: [w1253 w1256 w1280] -> w1240
              tunnel: w1238 -> [w1252 w1267 w1283]
              tunnel: [w1247 w1266 w1282] -> w1236
              tunnel: w1237 -> [_ w1265 w1281]
              tunnel: w1235 -> [_ w1254 _]
              tunnel: w1234 -> [_ _ w1278]
              tunnel: [T53 {"Gross Heating Value, Vol (Real, Dry)"=0.0, "Nitrogen Component Normalized Mole % (Dry)"=0.0, "Methane Component Normalized Mole % (Dry)"=0.0, "Carbon Dioxide Component Normalized Mole % (Dry)"=0.0, "Ethane Component Normalized Mole % (Dry)"=0.0, "Propane Component Normalized Mole % (Dry)"=0.0, "i-Pentane Component Normalized Mole % (Dry)"=0.0, "i-Butane Component Normalized Mole % (Dry)"=0.0, "n-Butane Component Normalized Mole % (Dry)"=0.0, "n-Pentane Component Normalized Mole % (Dry)"=0.0, "Hexane Component Normalized Mole % (Dry)"=0.0, "Heptane Component Normalized Mole % (Dry)"=0.0, "Gross Wobbe Index, Real(Dry)"=0.0, "Relative Density, Real(Dry)"=0.0, "Propylene Component Normalized Mole % (Dry)"=0.0, "C4 Olefins Component Normalized Mole % (Dry)"=0.0, "Water Component Normalized Mole % (Dry)"=0.0, "Gross Heating Value, Vol (Real, Sat)"=0.0, "Natural Gas Data"=[], "Propane Data"=[]} ("Inficon Data LP") w1254 w1278] -> w1233
              frame Default {
                n458 = Unbundle By Name(w1252) -> ("A Data Array"=w1251:string[][], "B Data Array"=w1250:string[][], "C Data Array"=w1249:string[][], "D Data Array"=w1248:string[][])
                n459 = Bundle By Name(cluster=w1252, "A Data Array"=w1251, "B Data Array"=w1250, "C Data Array"=w1249, "D Data Array"=w1248) -> (w1247:T88)
              }
              frame "CH4", "NatG-1", "NatG-2", "NatG-3" {
                n460 = Unbundle By Name(w1267) -> ("A Data Array"=w1261:string[][], "B Data Array"=w1262:string[][], "C Data Array"=w1263:string[][], "D Data Array"=w1264:string[][])
                n461 = Unbundle By Name(w1254) -> ("Natural Gas Data"=w1255)
                n462 = case shown="Default" w1265 {
                  tunnel: w1261 -> [w1269 w1277]
                  tunnel: w1262 -> [w1272 w1276]
                  tunnel: w1263 -> [w1271 w1275]
                  tunnel: w1264 -> [w1270 w1274]
                  tunnel: [w1273 w1277] -> w1260
                  tunnel: [w1272 w1276] -> w1259
                  tunnel: [w1271 w1275] -> w1258
                  tunnel: [w1270 w1274] -> w1257
                  tunnel: w1255 -> [w1268 _]
                  frame Default {
                    n463 = Build Array (concatenate)(w1269, w1268) -> (w1273:string[][])
                  }
                  frame "PRAT", "HEWH RLT" {
                  }
                }
                n464 = Bundle By Name(cluster=w1267, "A Data Array"=w1260, "B Data Array"=w1259, "C Data Array"=w1258, "D Data Array"=w1257) -> (w1266:T88)
              }
              frame "C3H8" {
                n465 = Unbundle By Name(w1283) -> ("A Data Array"=w1288:string[][], "B Data Array"=w1289:string[][], "C Data Array"=w1290:string[][], "D Data Array"=w1291:string[][])
                n466 = Unbundle By Name(w1278) -> ("Propane Data"=w1279)
                n467 = case shown="Default" w1281 {
                  tunnel: w1288 -> [w1293 w1301]
                  tunnel: w1289 -> [w1296 w1300]
                  tunnel: w1290 -> [w1295 w1299]
                  tunnel: w1291 -> [w1294 w1298]
                  tunnel: [w1297 w1301] -> w1287
                  tunnel: [w1296 w1300] -> w1286
                  tunnel: [w1295 w1299] -> w1285
                  tunnel: [w1294 w1298] -> w1284
                  tunnel: w1279 -> [w1292 _]
                  frame Default {
                    n468 = Build Array (concatenate)(w1293, w1292) -> (w1297:string[][])
                  }
                  frame "PRAT", "HEWH RLT" {
                  }
                }
                n469 = Bundle By Name(cluster=w1283, "A Data Array"=w1287, "B Data Array"=w1286, "C Data Array"=w1285, "D Data Array"=w1284) -> (w1282:T88)
              }
            }
            "Inficon Data" <- w1233
            n470 = call "HEWH HHV Notifier.vi"("Status"=UTILITY_Notifier."Set", "error in (no error)"=w1240, "Gas Measurment Data"=w1233, "name (unnamed)"="HHVData") -> ("error out"=w1239:errorcluster)  [unwired: 6 in, 1 out]
          }
          frame "Get Gas Data" {
            # "If Ritter Data is available,\ngo ahead and grab it"
            # "Get the Alicat Data"
            # "Acquire Gas Meter Data"
            n471 = call "Write String Array Units.vi"("Error In"=w1308) -> ("Alicate Gas Data - String"=w1305:string[][], "Error Out"=w1312:errorcluster)  [unwired: 13 in]
            n472 = Unbundle By Name(w1304) -> ("Core HEWH Data Input A.HEWH Specific DAQ.HEWH Data.HEWH Standard.TC 8"=w1303:dbl, "Core HEWH Data Input A.HEWH Specific DAQ.HEWH Data.HEWH Standard.PSI 1"=w1302:dbl)
            n473 = Unbundle By Name(w1304) -> ("A Data Array"=w1317:string[][], "B Data Array"=w1316:string[][], "C Data Array"=w1315:string[][], "D Data Array"=w1314:string[][], "Core HEWH Data Input A.LV Program"=w1313:T25)
            n474 = call "Ritter Write Data.vi"("Meter Type"="Meter Type", "error in (no error)"=w1312, "TC8"=w1303, "PSI 1"=w1302) -> ("String Data"=w1311:string[][], "error out"=w1307:errorcluster)  [unwired: 10 in]
            n475 = Build Array (concatenate)(w1305, w1311) -> (w1309:string[][])
            n476 = case shown="Default" w1313 {
              tunnel: w1317 -> [w1329 w1337]
              tunnel: w1316 -> [w1332 w1336]
              tunnel: w1315 -> [w1331 w1335]
              tunnel: w1314 -> [w1330 w1334]
              tunnel: [w1333 w1337] -> w1324
              tunnel: [w1332 w1336] -> w1323
              tunnel: [w1331 w1335] -> w1322
              tunnel: [w1330 w1334] -> w1321
              tunnel: w1309 -> [w1328 _]
              frame Default {
                n477 = Build Array (concatenate)(w1329, w1328) -> (w1333:string[][])
              }
              frame "PRAT", "HEWH RLT" {
              }
            }
            n478 = Unbundle By Name() -> ("Data Cluster"=w1306:T65)  [unwired: 1 in]
            "Gas Measurment Data" <- w1306
            n479 = Bundle By Name(cluster=w1304, "A Data Array"=w1324, "B Data Array"=w1323, "C Data Array"=w1322, "D Data Array"=w1321) -> (w1325:T88)
            n480 = call <vilib>:"Add State(s) to Queue__jki_lib_state_machine.vi"("State(s) in (\"\")"=w1327) -> ("States Out"=w1326:string)  [unwired: 14 in]
            n481 = call "HEWH Gas Notifier.vi"("Status"=UTILITY_Notifier."Set", "error in (no error)"=w1307, "Gas Measurment Data"=w1306, "name (unnamed)"="GasData") -> ("error out"=w1318:errorcluster)  [unwired: 6 in, 1 out]
          }
          frame "Get CO CO2" {
            # "Get Ultramat 23 Data (CO CO2)"
            n482 = Unbundle By Name(w1345) -> ("A Data Array"=w1349:string[][], "B Data Array"=w1348:string[][], "C Data Array"=w1347:string[][], "D Data Array"=w1346:string[][], "Core HEWH Data Input A.LV Program"=w1340:T25)
            n483 = call <vilib>:"Add State(s) to Queue__jki_lib_state_machine.vi"("State(s) in (\"\")"=w1352) -> ("States Out"=w1351:string)  [unwired: 14 in]
            n484 = local read item#-1() -> (w1339)
            "CO CO2 Data Array" <- w1339
            n485 = case shown="Default" w1340 {
              tunnel: w1349 -> [w1354 w1362]
              tunnel: w1348 -> [w1357 w1361]
              tunnel: w1347 -> [w1356 w1360]
              tunnel: w1346 -> [w1355 w1359]
              tunnel: [w1358 w1362] -> w1344
              tunnel: [w1357 w1361] -> w1343
              tunnel: [w1356 w1360] -> w1342
              tunnel: [w1355 w1359] -> w1341
              tunnel: w1339 -> [w1353 _]
              frame Default {
                n486 = Build Array (concatenate)(w1354, w1353) -> (w1358:string[][])
              }
              frame "PRAT", "HEWH RLT" {
              }
            }
            n487 = Bundle By Name(cluster=w1345, "A Data Array"=w1344, "B Data Array"=w1343, "C Data Array"=w1342, "D Data Array"=w1341) -> (w1350:T88)
          }
          frame "Get Vesta Data" {
            # "Get The Vesta Data"
            n488 = Unbundle By Name(w1372) -> ("A Data Array"=w1376:string[][], "B Data Array"=w1375:string[][], "C Data Array"=w1374:string[][], "D Data Array"=w1373:string[][], "Core HEWH Data Input A.LV Program"=w1367:T25)
            n489 = call <vilib>:"Add State(s) to Queue__jki_lib_state_machine.vi"("State(s) in (\"\")"=w1379) -> ("States Out"=w1378:string)  [unwired: 14 in]
            n490 = call "Resideo Gas Valve - Get Data.vi"("error in (no error)"=w1366) -> ("error out"=w1365:errorcluster, "Vesta Data Output"=→"Vesta Data Output":T66, "Vesta Data"=w1364:string[][])  [unwired: 8 in]
            n491 = case shown="\"PRAT\", \"HEWH RLT\"" w1367 {
              tunnel: w1376 -> [w1381 w1389]
              tunnel: w1375 -> [w1384 w1388]
              tunnel: w1374 -> [w1383 w1387]
              tunnel: w1373 -> [w1382 w1386]
              tunnel: [w1385 w1389] -> w1371
              tunnel: [w1384 w1388] -> w1370
              tunnel: [w1383 w1387] -> w1369
              tunnel: [w1382 w1386] -> w1368
              tunnel: w1364 -> [w1380 _]
              frame Default {
                n492 = Build Array (concatenate)(w1381, w1380) -> (w1385:string[][])
              }
              frame "PRAT", "HEWH RLT" {
              }
            }
            n493 = Bundle By Name(cluster=w1372, "A Data Array"=w1371, "B Data Array"=w1370, "C Data Array"=w1369, "D Data Array"=w1368) -> (w1377:T88)
          }
          frame "Data: Update Data Path A" {
            # "For RLT and PRAT, I create a new file each cycle. Prevents very large files"
            n494 = Unbundle By Name(w1391) -> ("Display Data (RLT).Station Label Display"=w1390:string)
            n495 = case shown="True" "New File Per CycA" {
              tunnel: w1392 -> [w1401 w1419]
              tunnel: w1396 -> [w1402 w1411]
              tunnel: [w1402 w1410] -> w1395
              tunnel: [w1399 w1408] -> w1394
              tunnel: w1390 -> [_ w1405]
              frame False {
                n496 = Bundle By Name(cluster=w1401, "File Locations A.New Summary Created"=FALSE) -> (w1399:T88)
              }
              frame True {
                # "I re-purposed this control. It now\ntriggers a header write in \"Data:\nSave\""
                # "I couldnt use a local to pass data due to UI Button"
                n497 = local read "Appliance Details A"() -> (w1404:T5)
                n498 = Unbundle By Name(w1419) -> ("Core HEWH Data Input A.LV Program"=w1403:T25, "File Locations A"=w1413:T3)
                n499 = property on="Cycle Count Display" class="DigNum (strict)"() -> ("Value"=w1406:i32)  [unwired: 2 in, 2 out]
                n500 = Unbundle By Name(w1404) -> ("Appliance Common.TR Number:"=w1417:string, "Appliance Common.Lab ID:"=w1416:string, "Appliance Common.Serial Number:"=w1415:string)
                n501 = Bundle By Name(cluster=T31 {"Appliance Details"={"FileVersionInfo"={"FileVersion"="", "ProductName"="", "InternalName"="", "CompanyName"="", "LegalCopyright"="", "FileDescription"=""}, "Dishwasher Info"={"Open Cup Weight (gm):"=0.0, "Auto Cup Weight (gm):"=0.0, "Detergent-Dish:"="", "Inlet Temperature-Dish:"="", "Cycle Mode-Dish:"="", "Unit Control-Dish:"="", "Manufacturer-Dish:"=""}, "Washer Info"={"Hot Water Temperature (Fahrenheit):"="", "Cold Water Temperature (Fahrenheit):"="", "Capacity (cu.ft):"=0.0, "Initial Cloth Weight:"=0.0, "Cloth Lot:"=0, "Model Family:"="", "Program Name:"="", "Cycle Selection:"="", "Wash Temperature:"="", "Rinse Temperature:"="", "Load Size:"=""}, "File Name Output Array"=[], "Calibration Output Array"=[], "Appliance Common"={"Engineer:"="", "Model Number:"="", "Serial Number:"="", "Comments:"="", "Station ID:"="", "Technician:"="", "TR Number:"="", "Lab ID:"="", "Voltage:"="", "Water Pressure (PSI):"="", "Test Date:"="", "Computer Name:"="", "IP Address:"="", "Ambient RH:"="", "Frequency:"="", "Build:"="", "Filename:"="", "Test Type:"="", "Load Run #:"=0, "Ambient Temperature (F):"="", "File Path:"=path "", "Cycles Per Year"=60}, "Water Heater"={"Heating Mode:"=""}, "Dryer"={"Heat Setting:"="", "Washer Water Temperature (60 ± 5°F):"=60, "Water Hardness (PPM):"=17, "Dryness Setting:"="", "Dryer Type:"="", "Exhaust:"="", "Drying Cycle:"="", "Load Type:"="", "Nominal Load Weight"="", "Dryer Initial IMC Data"={"Measured IMC (lbs)"=7.0, "Actual Initial RMC (%)"=7.0, "RMC (Desired %)"=100.0, "Bone Dry Wt(lbs)"=7.0, "Tolerance(%)"=5.0, "Actual Final RMC (%)"=0.0, "CEF (lbf/kWh)"=0.0, "Minimum Weight (lbf)"=0.0, "Average Weight (lbf)"=0.0, "Maximum Weight (lbf)"=0.0, "Measured IMC In Range?"=FALSE, "Moisture Reduction Factor"=55.5, "Field Use Factor"=1.04, "Empty Dryer Cold Weigth"=0.0, "Energy Standard"=enum."D2-Automatic Dryer", "Weight Cloth (lbs)"=0.0, "Relative Moisture Content (%)"=0.0, "Relative Moisture Content - Avg (%)"=0.0}}}, "Display Data (RLT)"={"Status Color"=0, "Serial Number Display"="", "Cycle Count Display"=0, "Station Label Display"="", "Current Run Start Time Display"=0.0, "Board ID Display"="", "RPM Display"=0, "Current Display"=0.0, "Current Path Display"=path "", "Saving Display"=FALSE, "Unit Type Display"=enum."", "Total Time On Display"=0.0, "UI Button"=FALSE}} ("Initialize.Washer In"), "Appliance Details.Appliance Common.TR Number:"=w1417, "Appliance Details.Appliance Common.Lab ID:"=w1416, "Appliance Details.Appliance Common.Serial Number:"=w1415, "Display Data (RLT).Station Label Display"=w1405, "Display Data (RLT).Cycle Count Display"=w1406) -> (w1414:T31)
                n502 = call "Save File Format All Folders.vi"("LV Program"=w1403, "error in (no error)"=w1411, "Initialize.Washer In"=w1414, "File Locations In"=w1413) -> ("error out"=w1410:errorcluster, "New File?"=w1407:bool, "File Locations Out"=w1412:T3)  [unwired: 5 in]
                n503 = Bundle By Name(cluster=w1419, "File Locations A"=w1412) -> (w1409:T88)
                n504 = Bundle By Name(cluster=w1409, "File Locations A.New Summary Created"=w1407) -> (w1408:T88)
              }
            }
            n505 = call <vilib>:"Add State(s) to Queue__jki_lib_state_machine.vi"("State(s) in (\"\")"=w1398) -> ("States Out"=w1397:string)  [unwired: 14 in]
          }
          frame "Data: Update Data Path B" {
            n506 = Unbundle By Name(w1421) -> ("Display Data (RLT).Station Label Display"=w1420:string)
            n507 = case shown="True" "New File Per CycB" {
              tunnel: w1426 -> [w1431 w1449]
              tunnel: w1425 -> [w1432 w1441]
              tunnel: [w1432 w1440] -> w1424
              tunnel: [w1430 w1438] -> w1423
              tunnel: w1420 -> [_ w1434]
              frame False {
                n508 = Bundle By Name(cluster=w1431, "File Locations B.New Summary Created"=FALSE) -> (w1430:T88)
              }
              frame True {
                # "I re-purposed this control. It now\ntriggers a header write in \"Data:\nSave\""
                # "I couldnt use a local to pass data due to UI Button"
                n509 = local read "Appliance Details B"() -> (w1435:T5)
                n510 = Unbundle By Name(w1449) -> ("Core HEWH Data Input B.LV Program"=w1433:T25, "File Locations B"=w1444:T3)
                n511 = Unbundle By Name(w1435) -> ("Appliance Common.TR Number:"=w1447:string, "Appliance Common.Lab ID:"=w1446:string, "Appliance Common.Serial Number:"=w1445:string)
                n512 = property on="Cycle Count Display" class="DigNum (strict)"() -> ("Value"=w1436:i32)  [unwired: 2 in, 2 out]
                n513 = Bundle By Name(cluster=T31 {"Appliance Details"={"FileVersionInfo"={"FileVersion"="", "ProductName"="", "InternalName"="", "CompanyName"="", "LegalCopyright"="", "FileDescription"=""}, "Dishwasher Info"={"Open Cup Weight (gm):"=0.0, "Auto Cup Weight (gm):"=0.0, "Detergent-Dish:"="", "Inlet Temperature-Dish:"="", "Cycle Mode-Dish:"="", "Unit Control-Dish:"="", "Manufacturer-Dish:"=""}, "Washer Info"={"Hot Water Temperature (Fahrenheit):"="", "Cold Water Temperature (Fahrenheit):"="", "Capacity (cu.ft):"=0.0, "Initial Cloth Weight:"=0.0, "Cloth Lot:"=0, "Model Family:"="", "Program Name:"="", "Cycle Selection:"="", "Wash Temperature:"="", "Rinse Temperature:"="", "Load Size:"=""}, "File Name Output Array"=[], "Calibration Output Array"=[], "Appliance Common"={"Engineer:"="", "Model Number:"="", "Serial Number:"="", "Comments:"="", "Station ID:"="", "Technician:"="", "TR Number:"="", "Lab ID:"="", "Voltage:"="", "Water Pressure (PSI):"="", "Test Date:"="", "Computer Name:"="", "IP Address:"="", "Ambient RH:"="", "Frequency:"="", "Build:"="", "Filename:"="", "Test Type:"="", "Load Run #:"=0, "Ambient Temperature (F):"="", "File Path:"=path "", "Cycles Per Year"=60}, "Water Heater"={"Heating Mode:"=""}, "Dryer"={"Heat Setting:"="", "Washer Water Temperature (60 ± 5°F):"=60, "Water Hardness (PPM):"=17, "Dryness Setting:"="", "Dryer Type:"="", "Exhaust:"="", "Drying Cycle:"="", "Load Type:"="", "Nominal Load Weight"="", "Dryer Initial IMC Data"={"Measured IMC (lbs)"=7.0, "Actual Initial RMC (%)"=7.0, "RMC (Desired %)"=100.0, "Bone Dry Wt(lbs)"=7.0, "Tolerance(%)"=5.0, "Actual Final RMC (%)"=0.0, "CEF (lbf/kWh)"=0.0, "Minimum Weight (lbf)"=0.0, "Average Weight (lbf)"=0.0, "Maximum Weight (lbf)"=0.0, "Measured IMC In Range?"=FALSE, "Moisture Reduction Factor"=55.5, "Field Use Factor"=1.04, "Empty Dryer Cold Weigth"=0.0, "Energy Standard"=enum."D2-Automatic Dryer", "Weight Cloth (lbs)"=0.0, "Relative Moisture Content (%)"=0.0, "Relative Moisture Content - Avg (%)"=0.0}}}, "Display Data (RLT)"={"Status Color"=0, "Serial Number Display"="", "Cycle Count Display"=0, "Station Label Display"="", "Current Run Start Time Display"=0.0, "Board ID Display"="", "RPM Display"=0, "Current Display"=0.0, "Current Path Display"=path "", "Saving Display"=FALSE, "Unit Type Display"=enum."", "Total Time On Display"=0.0, "UI Button"=FALSE}} ("Initialize.Washer In"), "Appliance Details.Appliance Common.TR Number:"=w1447, "Appliance Details.Appliance Common.Lab ID:"=w1446, "Appliance Details.Appliance Common.Serial Number:"=w1445, "Display Data (RLT).Station Label Display"=w1434, "Display Data (RLT).Cycle Count Display"=w1436) -> (w1443:T31)
                n514 = call "Save File Format All Folders.vi"("LV Program"=w1433, "error in (no error)"=w1441, "Initialize.Washer In"=w1443, "File Locations In"=w1444) -> ("error out"=w1440:errorcluster, "New File?"=w1437:bool, "File Locations Out"=w1442:T3)  [unwired: 5 in]
                n515 = Bundle By Name(cluster=w1449, "File Locations B"=w1442) -> (w1439:T88)
                n516 = Bundle By Name(cluster=w1439, "File Locations B.New Summary Created"=w1437) -> (w1438:T88)
              }
            }
